vi "network_recv.vi"(6 "Reset":bool, 9 "Network In":sgl[](array[numeric]), 10 "Goal position in":sgl[][](array[numeric]), 11 "Recv UDP Conn":refnum<k16>) -> (1 "Network Out":sgl[](array[numeric]), 2 "Goal position out":sgl[][](array[numeric]))   [LabVIEW 2014]
panel:
  in  "Stuff it":bool
  in  "Stuff packet":sgl[](array[numeric])
  out "Packets received":u32
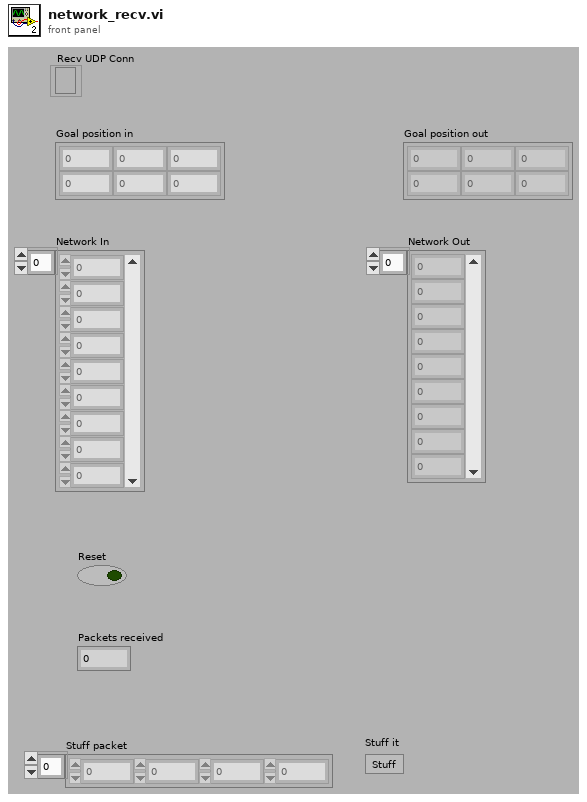
[diagram p1: front panel]
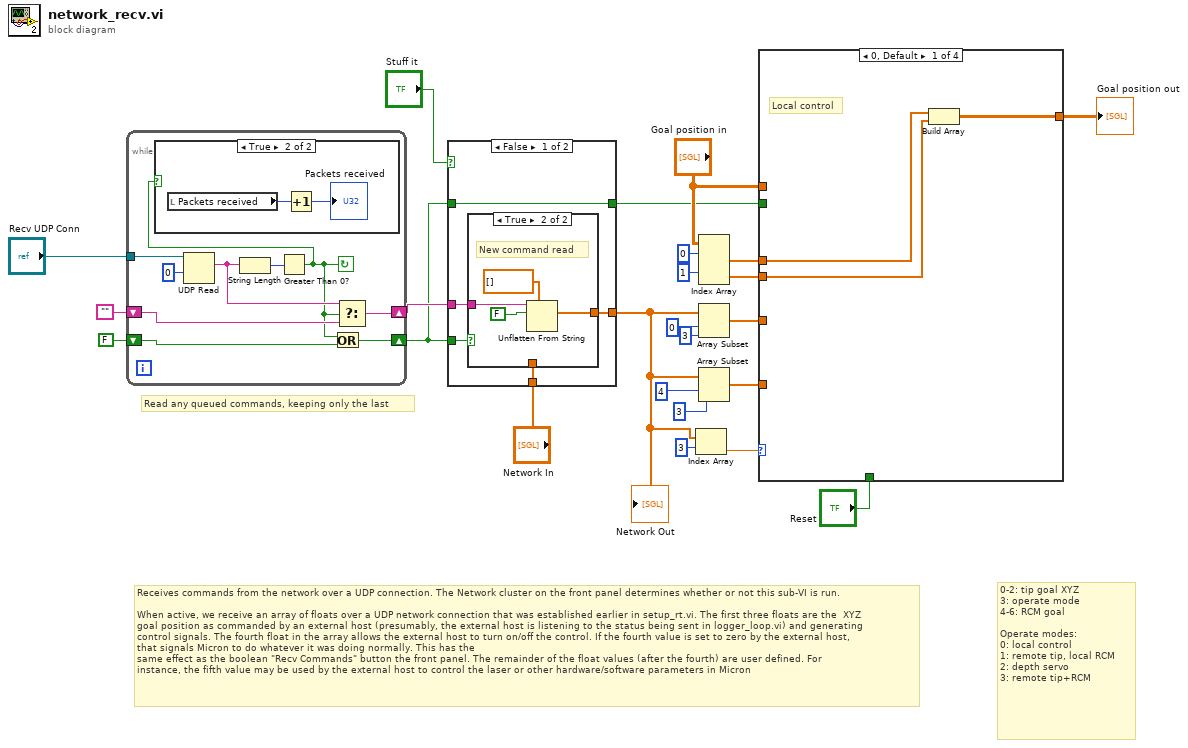
[diagram p0: block diagram]
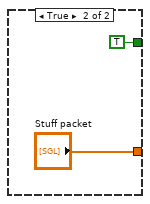
[diagram p3: hidden frame]
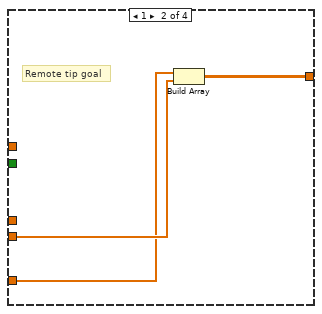
[diagram p4: hidden frame]
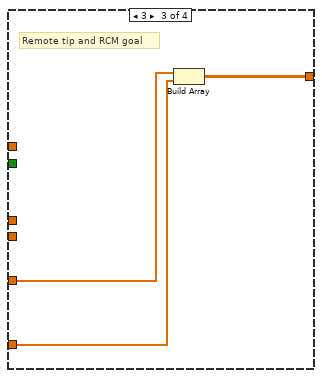
[diagram p5: hidden frame]
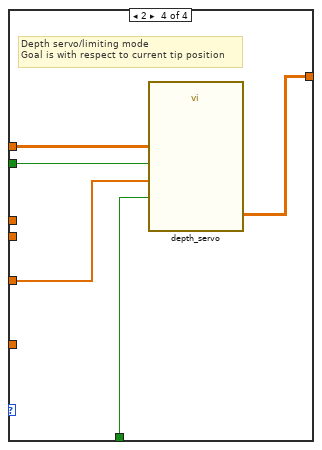
[diagram p6: hidden frame]
diagram:
  # "0-2: tip goal XYZ\n3: operate mode\n4-6: RCM goal\n\nOperate modes:\n0: local control\n1: remote tip, local RCM\n2: depth servo\n3: remote tip+RCM"
  # "Read any queued commands, keeping only the last"
  # "Receives commands from the network over a UDP connection. The Network cluster on the front panel determines whether or not this sub-VI is run.\n\nWhen active, we receive an array of floats over a UDP network connection that was established earlier in setup_rt.vi. The first three floats are the  XYZ\ngoal position as commanded by an external host (presumably, the external host is listening to the status being sent in logger_loop.vi) and generating\ncontrol signals. The fourth float in the array allows the external host to turn on/off the control. If the fourth value is set to zero by the external host, \nthat signals Micron to do whatever it was doing normally. This has the \nsame effect as the boolean \"Recv Commands\" button the front panel. The remainder of the float values (after the fourth) are user defined. For\ninstance, the fifth value may be used by the external host to control the laser or other hardware/software parameters in Micron"
  n1 = while {
    tunnel: "Recv UDP Conn" -> [w32]
    shift-right: [w28] -> w24
    shift-left: "" -> [w30]
    shift-right: [w26] -> w6
    shift-left: FALSE -> [w27]
    stop <- w25 continue-if-true
    n2 = UDP Read(connection ID=w32, timeout ms (25000)=0) -> (data out=w29:string)  [unwired: 1 in, 5 out]
    n3 = String Length(string=w29) -> (length=w31:i32)
    n4 = Greater Than 0?(x=w31) -> (x > 0?=w25:bool)
    n5 = case shown="True" w25 {
      frame False {
      }
      frame True {
        n6 = local read "Packets received"() -> (w35:u32)
        n7 = Increment(x=w35) -> (x+1=→"Packets received":u32)
      }
    }
    n8 = Or(x=w25, y=w27) -> (x .or. y?=w26:bool)
    n9 = Select(t=w29, s=w25, f=w30) -> (s? t:f=w28:string)
  }
  n10 = case shown="False" "Stuff it" {
    tunnel: w24 -> [w40 _]
    tunnel: [w39 "Stuff packet"] -> w2
    tunnel: "Network In" -> [w38 _]
    tunnel: w6 -> [w37 _]
    tunnel: w6 -> [w36 _]
    tunnel: [w36 TRUE] -> w5
    frame False {
      n11 = case shown="True" w37 {
        tunnel: [w41 w45] -> w39
        tunnel: w40 -> [_ w44]
        tunnel: w38 -> [w41 _]
        frame False {
          # "No new command"
        }
        frame True {
          # "New command read"
          n12 = Unflatten From String(type=sgl[] [], binary string=w44, data includes array or string size? (T)=FALSE) -> (value=w45:sgl[])  [unwired: 1 in, 3 out]
        }
      }
    }
    frame True {
    }
  }
  "Network Out" <- w2
  n13 = Index Array(array=w2, index=3 ("t")) -> (element=w11:sgl)
  n14 = Index Array(array="Goal position in", index (row) #1=0 ("index (row)"), index (row) #2=1 ("index (row)")) -> (element #1=w12:sgl[], element #2=w14:sgl[])  [unwired: 2 in]
  n15 = Array Subset(array=w2, index=0 ("t"), length=3 ("t")) -> (w10:sgl[])
  n16 = Array Subset(array=w2, index=4 ("t"), length=3 ("t")) -> (w1:sgl[])
  n17 = case shown="0, Default" w11 {
    tunnel: w14 -> [w50 w53 _ _]
    tunnel: [w49 w52 w56 w57] -> w13
    tunnel: w12 -> [w48 _ _ _]
    tunnel: w10 -> [_ w51 w55 w60]
    tunnel: w5 -> [_ _ _ w61]
    tunnel: "Reset" -> [_ _ _ w59]
    tunnel: "Goal position in" -> [_ _ _ w58]
    tunnel: w1 -> [_ _ w54 _]
    frame 0, Default {
      # "Local control"
      n18 = Build Array(w48, w50) -> (w49:sgl[][])
    }
    frame 1 {
      # "Remote tip goal"
      n19 = Build Array(w51, w53) -> (w52:sgl[][])
    }
    frame 3 {
      # "Remote tip and RCM goal"
      n20 = Build Array(w55, w54) -> (w56:sgl[][])
    }
    frame 2 {
      # "Depth servo/limiting mode\nGoal is with respect to current tip position"
      n21 = call "depth_servo.vi"("Current depth"=w60, "New command"=w61, "Goal position in"=w58, "Reset"=w59) -> ("Goal position out"=w57:sgl[][])  [unwired: 7 in]
    }
  }
  "Goal position out" <- w13
